vi "simple network stream trial with auto reconnect.vi"() -> ()   [LabVIEW 2018]
uses:
  <resource>/objmgr/ni.dex.rc
panel:
  in  "Stop":bool
  in  "disconnect":bool
  in  "reconnect":bool
  out "read message":string
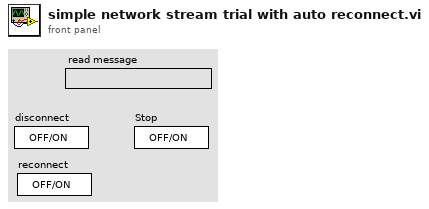
[diagram p1: front panel]
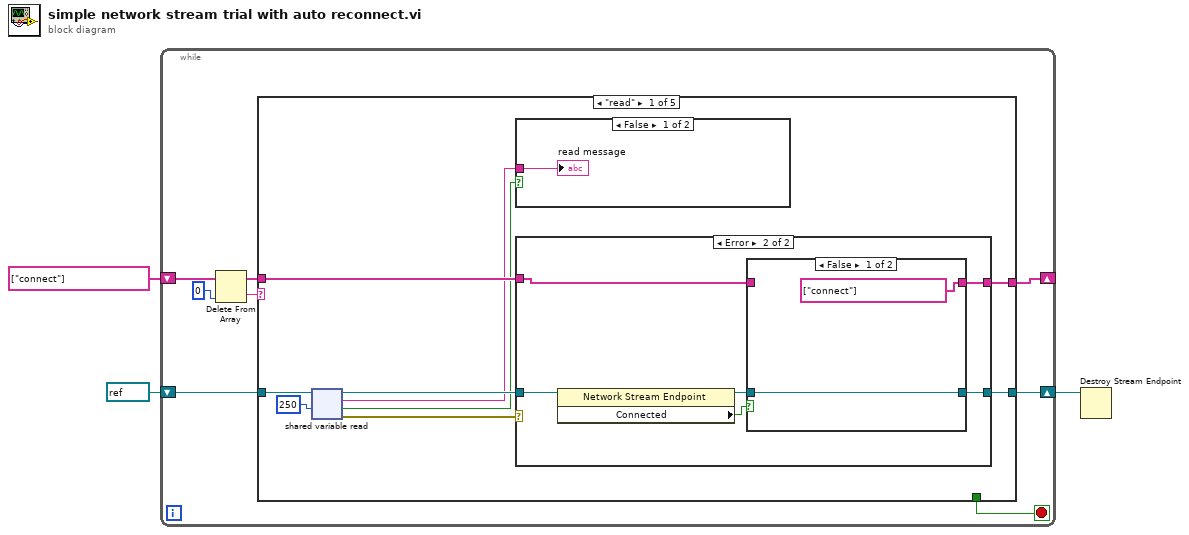
[diagram p0: block diagram]
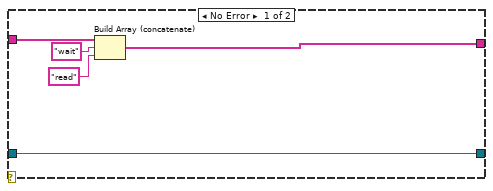
[diagram p3: hidden frame]
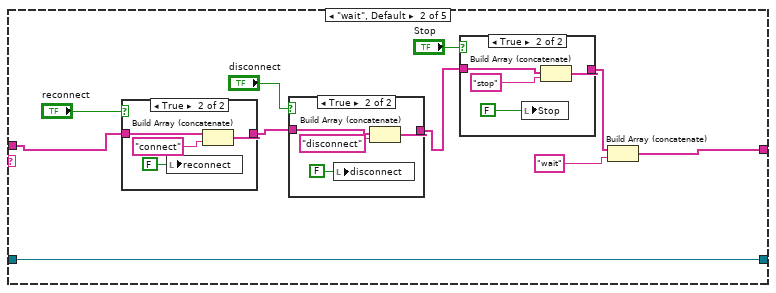
[diagram p5: hidden frame]
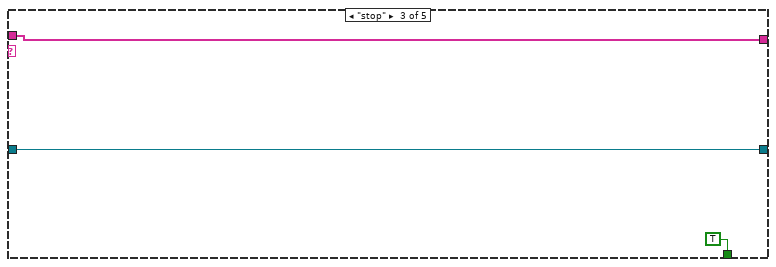
[diagram p9: hidden frame]
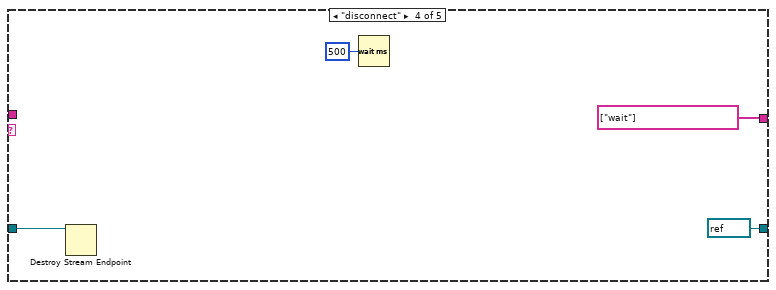
[diagram p10: hidden frame]
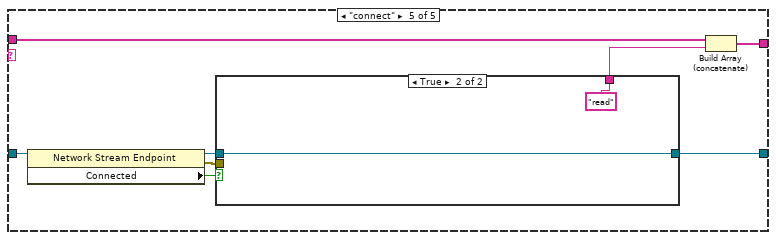
[diagram p11: hidden frame]
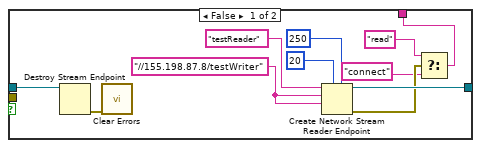
[diagram p12: hidden frame]
diagram:
  n1 = while {
    shift-right: [w7] -> _
    shift-left: string[] ["connect"] -> [w11]
    shift-right: [w6] -> w1
    shift-left: refnum<k21> refnum ("reader name") -> [w5]
    stop <- w4 stop-if-true
    n2 = Delete From Array(array=w11, index=0) -> (deleted portion=w9:string, array with subset deleted=w8:string[])  [unwired: 1 in]
    n3 = case shown="\"read\"" w9 {
      tunnel: w8 -> [w15 w42 w64 _ w72]
      tunnel: [w14 w46 w64 string[] ["wait"] w71] -> w7
      tunnel: [w16 w44 w63 refnum<k21> refnum ("reader name") w76] -> w6
      tunnel: w5 -> [w20 w44 w63 w68 w75]
      tunnel: [_ _ TRUE _ _] -> w4
      frame "read" {
        n4 = shared-variable-read(w20, 250 ("timeout ms (-1)")) -> (w17:refnum<k21>, w18:errorcluster, w12:bool, w13:string)  [unwired: 1 in]
        n5 = case shown="False" w12 {
          tunnel: w13 -> [w21 _]
          frame False {
            "read message" <- w21
          }
          frame True {
          }
        }
        n6 = case shown="Error" w18 {
          tunnel: w17 -> [w23 w32]
          tunnel: [w23 w29] -> w16
          tunnel: w15 -> [w25 w28]
          tunnel: [w24 w27] -> w14
          frame No Error {
            n7 = Build Array (concatenate)(w25, "wait" ("reader name"), "read" ("reader name")) -> (w24:string[])
          }
          frame Error {
            n8 = property class="Network Stream Endpoint"(reference=w32) -> (reference out=w30:refnum<k21>, "Connected"=w31:bool)  [unwired: 1 in, 1 out]
            n9 = case shown="False" w31 {
              tunnel: w30 -> [w33 w36]
              tunnel: [w33 w36] -> w29
              tunnel: w28 -> [_ w35]
              tunnel: [string[] ["connect"] w35] -> w27
              frame False {
              }
              frame True {
              }
            }
          }
        }
      }
      frame "wait", Default {
        n10 = case shown="True" "reconnect" {
          tunnel: w42 -> [w57 w61]
          tunnel: [w57 w60] -> w41
          frame False {
          }
          frame True {
            n11 = local write "reconnect"(FALSE ("reconnect")) -> ()
            n12 = Build Array (concatenate)(w61, "connect" ("String")) -> (w60:string[])
          }
        }
        n13 = case shown="True" "disconnect" {
          tunnel: [w52 w56] -> w39
          tunnel: w41 -> [w52 w54]
          frame False {
          }
          frame True {
            n14 = local write "disconnect"(FALSE ("disconnect")) -> ()
            n15 = Build Array (concatenate)(w54, "disconnect" ("String")) -> (w56:string[])
          }
        }
        n16 = case shown="True" "Stop" {
          tunnel: [w47 w51] -> w38
          tunnel: w39 -> [w47 w49]
          frame False {
          }
          frame True {
            n17 = local write "Stop"(FALSE ("disconnect")) -> ()
            n18 = Build Array (concatenate)(w49, "stop" ("String")) -> (w51:string[])
          }
        }
        n19 = Build Array (concatenate)(w38, "wait" ("String")) -> (w46:string[])
      }
      frame "stop" {
      }
      frame "disconnect" {
        n20 = Destroy Stream Endpoint(11:w68) -> ()  [unwired: 1 in, 1 out]
        n21 = Wait (ms)(milliseconds to wait=u32 500) -> ()  [unwired: 1 out]
      }
      frame "connect" {
        n22 = property class="Network Stream Endpoint"(reference=w75) -> (reference out=w73:refnum<k21>, error out=w70:errorcluster, "Connected"=w74:bool)  [unwired: 1 in]
        n23 = case shown="True" w74 {
          tunnel: [w85 w89] -> w76
          tunnel: w73 -> [w84 w89]
          tunnel: w70 -> [_ _]
          tunnel: [w77 "read" ("reader name")] -> w69
          frame False {
            w86 = "//155.198.87.8/testWriter" ("writer url")
            n24 = Destroy Stream Endpoint(11:w84) -> (0:w83:errorcluster)  [unwired: 1 in]
            n25 = call <vilib>:"Clear Errors.vi"("error in (no error)"=w83) -> ()  [unwired: 5 in, 2 out]
            n26 = Create Network Stream Reader Endpoint(5:250 ("timeout in ms (-1)"), 7:20 ("reader buffer size"), 9:w86, 10:w86, 11:"testReader" ("reader name")) -> (0:w80:errorcluster, 3:w85:refnum<k21>)  [unwired: 2 in]
            n27 = Select(t="read" ("reader name"), s=w80, f="connect" ("reader name")) -> (s? t:f=w77:string)
          }
          frame True {
          }
        }
        n28 = Build Array (concatenate)(w72, w69) -> (w71:string[])
      }
    }
  }
  n29 = Destroy Stream Endpoint(11:w1) -> ()  [unwired: 1 in, 1 out]
